vi "Send Timer Update Display.vi"(7 "Message Priority (Normal)":T1=enum."Normal", 8 "error in (no error)":errorcluster, 9 "Current Time":dbl, 10 "Starting Time":dbl, 11 "Message Enqueuer":refnum<class "Message Enqueuer.lvclass">) -> (0 "error out":errorcluster, 3 "Message Enqueuer out":refnum<class "Message Enqueuer.lvclass">)   [LabVIEW 2024, in "Controller.lvlib" / "Timer Update Display Msg.lvclass"]
doc: "This VI sends the message to an actor."
uses:
  Timer Update Display Msg.lvclass
  <vilib>/ActorFramework/Message Enqueuer/Message Enqueuer.lvclass
  <vilib>/ActorFramework/Message Enqueuer/Message Priority.ctl
  Applications/National Instruments/LabVIEW 2024 64-bit/vi.lib/ActorFramework/Message/Message.lvclass
  Timer Update Display Msg.lvclass/Timer Update Display Msg.ctl
  <vilib>/ActorFramework/Message Enqueuer/Message Enqueuer.lvclass/Message Enqueuer.ctl
  <vilib>/ActorFramework/Message Priority Queue/Priority Enqueue.vi
  Users/elijahkerry/challenge-of-champions/Controller/Controller Messages/Timer Update Display Msg/Timer Update Display Msg.lvclass
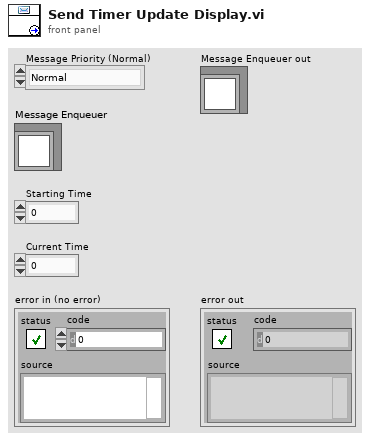
[diagram p1: front panel]
types:
  T1 = typedef "Actor Framework.lvlib/Message Enqueuer.lvclass/Message Priority.ctl" = enum16{"Low", "Normal", "High"}
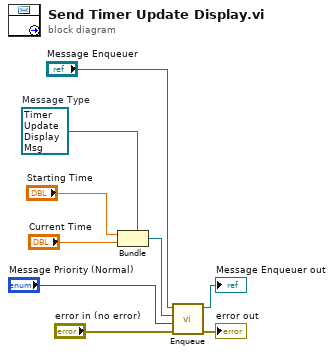
[diagram p0: block diagram]
diagram:
  w6 = refnum<class "Timer Update Display Msg.lvclass"> refnum  # Message Type
  n1 = Bundle(cluster=w6, "Starting Time", "Current Time") -> (w5:refnum<class "Timer Update Display Msg.lvclass">)
  n2 = call <vilib>:"Enqueue.vi"("error in (no error)"="error in (no error)", "Message Priority (Normal)"="Message Priority (Normal)", "Message"=w5, "Message Enqueuer in"="Message Enqueuer") -> ("error out"=→"error out":errorcluster, "Message Enqueuer in"=→"Message Enqueuer out":refnum<class "Message Enqueuer.lvclass">)  [unwired: 6 in]
